vi "Load_Build_Type.vi"(8 "error in (no error)":errorcluster, 11 "buildObject":T1) -> (0 "error out":errorcluster, 3 "AB_Build out":refnum<class "AB_Build.lvclass">)   [LabVIEW 2020, in "AB_Build.lvclass"]
uses:
  <vilib>/AppBuilder/AB_Classes/Build/AB_Build.lvclass
  <resource>/Framework/Providers/API/ItemRef.ctl
  <vilib>/AppBuilder/AB_Classes/Build/AB_Build.lvclass/AB_Build.ctl
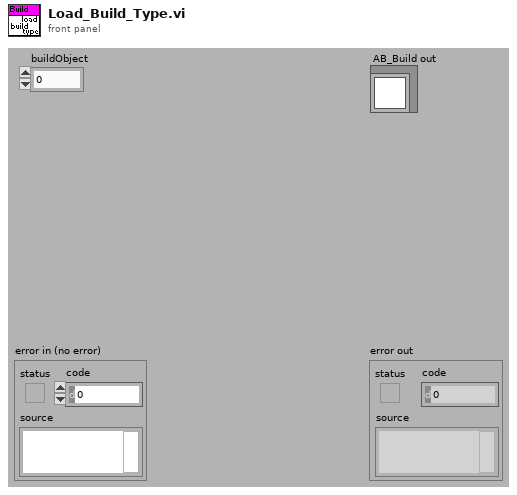
[diagram p1: front panel]
types:
  T1 = typedef "ItemRef.ctl" = u64
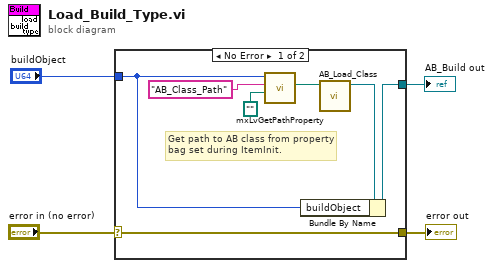
[diagram p0: block diagram]
diagram:
  n1 = case shown="No Error" "error in (no error)" {
    selector: "error in (no error)" -> [w11 w12]
    tunnel: [w11 w12] -> w3
    tunnel: [w10 _] -> w2
    tunnel: "buildObject" -> [w8 _]
    frame No Error {
      # "Get path to AB class from property bag set during ItemInit."
      n2 = call <resource>:"mxLvGetPathProperty.vi"("Default Path"=path "", "Tag"="AB_Class_Path", "Item"=w8) -> ("Path"=w7:path)  [unwired: 6 in, 2 out]
      n3 = call <vilib>:"AB_Load_Class.vi"("AB_Class path"=w7) -> ("AB_Build out"=w9:refnum<class "AB_Build.lvclass">)  [unwired: 9 in, 1 out]
      n4 = Bundle By Name(cluster=w9, "buildObject"=w8) -> (w10:refnum<class "AB_Build.lvclass">)
    }
    frame Error {
    }
  }
  "error out" <- w3
  "AB_Build out" <- w2
